vi "Aperture Cal.vi"(1 "Calibration Axis Info (Aperture Calibration)":T4={"Origin Pixel"={"X"=227.0, "Y"=1000.0}, "X Axis Pixel"={"X"=276.9972, "Y"=1000.52985}, "Axis Reference"=1} {"Axis Reference" items=["Direct", "Indirect"]}) -> (27 "error out":errorcluster)   [LabVIEW 2018]
uses:
  <vilib>/userdefined/High Color/IMAQdx.ctl
  <vilib>/vision/Image Controls.llb/Vision Info Type2.ctl
  <vilib>/vision/NI_Vision_Development_Module.lvlib
  <vilib>/vision/driver/NI_Vision_Acquisition_Software.lvlib
panel:
  out "x*y":dbl
  out "x-y":u16
  in  "BCG":T1 {"GAMMA" format="%_3f"}
  in  "Boolean":bool
  in  "PIXEL CALIBRATION":T2={"XSTEP SIZE"=5.7150000000000025, "YSTEP SIZE"=6.25, "UNITS"=2} {"UNITS" items=["Undefined", "Angstroms", "Microns"]; "YSTEP SIZE" format="%_4g"; "XSTEP SIZE" format="%_4g"}
  out "Image":T3(plugin-control)
  out "Line Profile Graph":u8[](graph) caption="Line Profile"
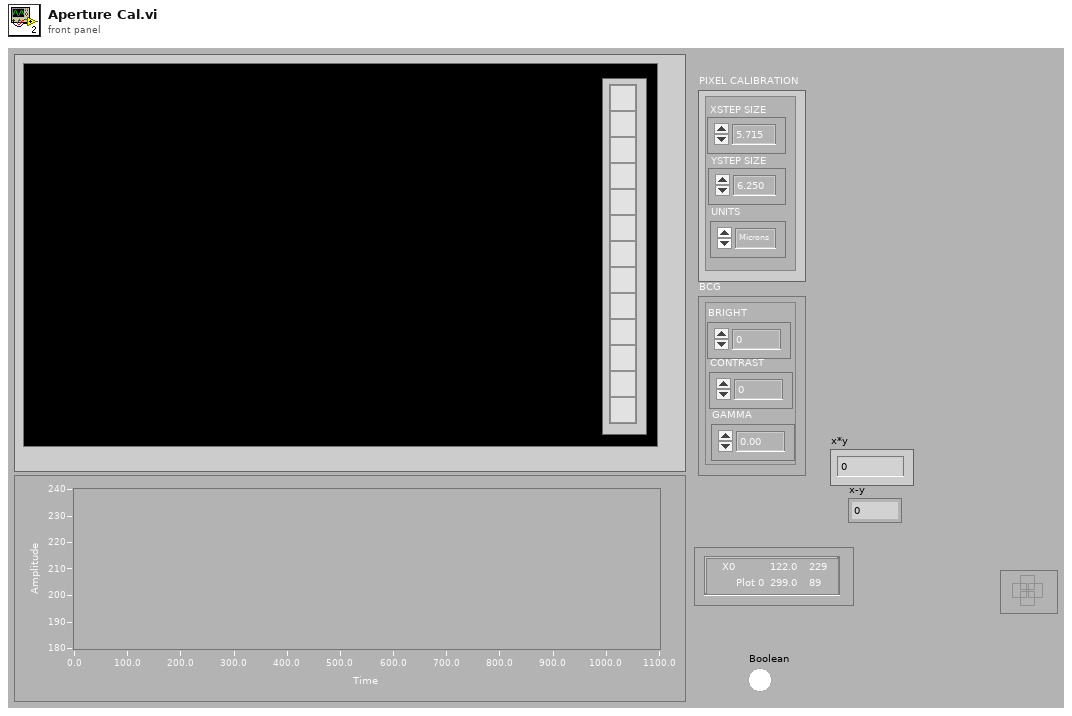
[diagram p1: front panel]
types:
  T1 = cluster{"BRIGHT":dbl, "CONTRAST":dbl, "GAMMA":dbl}
  T2 = cluster{"XSTEP SIZE":dbl, "YSTEP SIZE":dbl, "UNITS":u16}
  T3 = typedef "IMAQ Image.ctl" = refnum<image>
  T4 = cluster{"Origin Pixel":cluster{"X":sgl, "Y":sgl}, "X Axis Pixel":cluster{"X":sgl, "Y":sgl}, "Axis Reference":u32}
  T5 = typedef "IMAQdx.ctl" = refnum<k21>
  T6 = typedef "Vision Info Type2.ctl" = u32
  T7 = cluster{"Global Rectangle":i32[], "Contours":cluster{"Contour Type":u32, "ROI Type":u32, "Points":i32[]}[]}
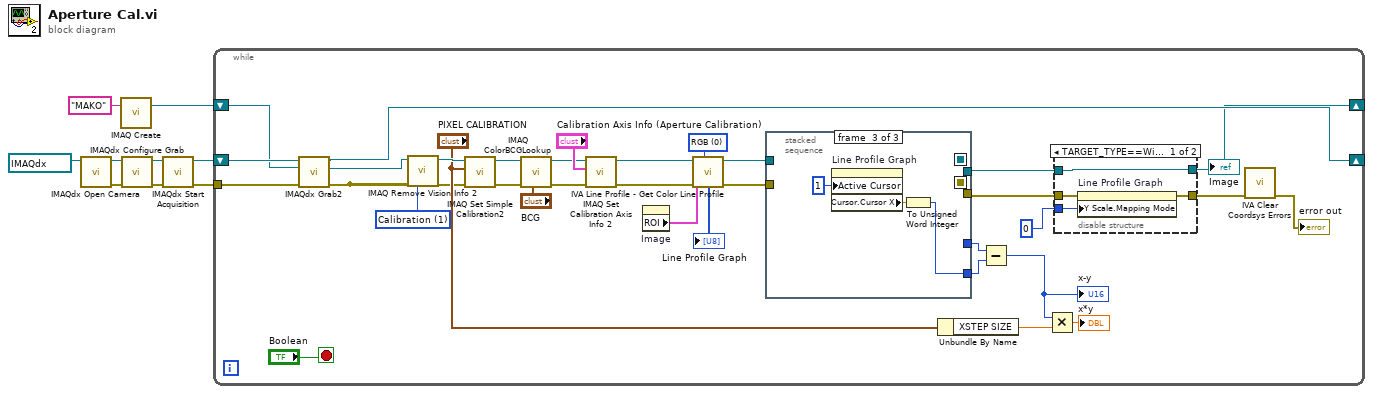
[diagram p0: block diagram]
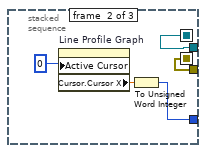
[diagram p3: hidden frame]
diagram:
  n1 = call <vilib>:"IMAQdx Open Camera.vi"("Session In"=T5 "MAKO") -> ("error out"=w6:errorcluster, "Session Out"=w8:T5)  [unwired: 9 in]
  n2 = call "IMAQ Create"("Image Name"="MAKO") -> ("New Image"=w1:T3)  [unwired: 4 in, 1 out]
  n3 = call <vilib>:"IMAQdx Configure Grab.vi"("error in"=w6, "Session In"=w8) -> ("error out"=w4:errorcluster, "Session Out"=w7:T5)  [unwired: 8 in]
  n4 = call <vilib>:"IMAQdx Start Acquisition.vi"("error in"=w4, "Session In"=w7) -> ("error out"=w3:errorcluster, "Session Out"=w5:T5)  [unwired: 8 in]
  n5 = while {
    tunnel: w3 -> [w16]
    shift-right: [w12] -> _
    shift-left: w5 -> [w15]
    shift-right: [w10] -> _
    shift-left: w1 -> [w11]
    stop <- "Boolean" stop-if-true
    w40 = u16 0 items=["RGB", "HSL", "HSV", "HSI"] ("Color Mode")
    w43 = T6 1 items=["Any", "Calibration", "Overlay", "Grayscale Template", "Color Template", "Geometric Template", "Custom Data", "Golden Template", "Geometric Template 2", "Contour Data", "Camera Model"] ("Vision Info")
    n6 = call <vilib>:"IMAQdx Grab2.vi"("error in"=w16, "Image In"=w11, "Session In"=w15) -> ("error out"=w13:errorcluster, "Image Out"=w14:T3, "Session Out"=w12:T5)  [unwired: 5 in, 1 out]
    n7 = call "IMAQ Remove Vision Info 2"("error in (no error)"=w13, "Vision Info"=w43, "Image"=w14) -> ("Image Out"=w42:T3)  [unwired: 8 out]
    n8 = call "IMAQ Set Simple Calibration2"("error in (no error)"=w13, "Pixel Distances"="PIXEL CALIBRATION", "Image"=w42) -> ("error out"=w30:errorcluster, "Calibration Template Image"=w32:T3)  [unwired: 2 in, 5 out]
    n9 = call "IMAQ ColorBCGLookup"("Green BCG Values"="BCG", "error in (no error)"=w30, "Image Src"=w32) -> ("error out"=w29:errorcluster, "Image Dst Out"=w31:T3)  [unwired: 4 in, 3 out]
    n10 = call-poly "IMAQ Set Calibration Axis Info 2"("error in (no error)"=w29, "Calibration Axis Info"="Calibration Axis Info (Aperture Calibration)", "Calibration Template Image In"=w31) -> ("error out"=w38:errorcluster, "Calibration Template Image Out"=w39:T3)  [unwired: 7 out]
    n11 = property on="Image" class="ImageControl"() -> ("ROI"=w27:T7)  [unwired: 2 in, 2 out]
    n12 = call <vilib>:"IVA Line Profile - Get Color Line Profile.vi"("Color Mode"=w40, "error in (no error)"=w38, "ROI Descriptor"=w27, "Image In"=w39) -> ("error out"=w23:errorcluster, "Green or Sat Pixels"=→"Line Profile Graph":u8[], "Image Out"=w25:T3)  [unwired: 5 out]
    n13 = stacked-sequence {
      seq-local: [w45 _ _] -> [_ w47 _]
      seq-local: [w44 _ _] -> [_ w46 _]
      tunnel: w25 -> [w45 _ _]
      tunnel: w23 -> [w44 _ _]
      tunnel: [_ w47 _] -> w26
      tunnel: [_ w46 _] -> w24
      tunnel: [_ w48 _] -> w22
      tunnel: [_ _ w51] -> w21
      frame #0 {
      }
      frame #1 {
        n14 = property on="Line Profile Graph" class="WFGraph (strict)"("Active Cursor"=u32 0) -> ("Cursor.Cursor X"=w49:dbl)  [unwired: 2 in, 2 out]
        n15 = To Unsigned Word Integer(number=w49) -> (unsigned 16bit integer=w48:u16)
      }
      frame #2 {
        n16 = property on="Line Profile Graph" class="WFGraph (strict)"("Active Cursor"=u32 1) -> ("Cursor.Cursor X"=w52:dbl)  [unwired: 2 in, 2 out]
        n17 = To Unsigned Word Integer(number=w52) -> (unsigned 16bit integer=w51:u16)
      }
    }
    n18 = Unbundle By Name("PIXEL CALIBRATION") -> ("XSTEP SIZE"=w18:dbl)
    n19 = Subtract(x=w22, y=w21) -> (x-y=w20:u16)
    "x-y" <- w20
    n20 = Multiply(x=w20, y=w18) -> (x*y=→"x*y":dbl)
    n21 = disable-structure "Conditional Disable Structure" shown="TARGET_TYPE==Windows" {
      disable-tunnel: w24 -> [w57 w58]
      disable-tunnel: [w56 w58] -> w36
      disable-tunnel: w26 -> [w55 w59]
      disable-tunnel: [w55 w59] -> w10
      disable-tunnel: u8 0 ("Y Scale.Mapping Mode") -> [w54 _]
      frame condition #0 (active) {
        n22 = property on="Line Profile Graph" class="WFGraph (strict)"(error in=w57, "Y Scale.Mapping Mode"=w54) -> (error out=w56:errorcluster)  [unwired: 1 in, 1 out]
      }
      frame condition #1 {
      }
    }
    "Image" <- w10
    n23 = call <vilib>:"IVA Clear Coordsys Errors.vi"("error in (no error)"=w36) -> ("error out"=→"error out":errorcluster)  [unwired: 10 in]
  }
